vi "Physical Constant Menu.vi"() -> ()   [LabVIEW 2013]
panel:
  in  "Minimum Z Extension (nm)":dbl
  in  "Maximum Z Extension (nm)":dbl
  in  "Z Piezo Response (nm/V)":dbl
  in  "Minimum Y Extension (nm)":dbl
  in  "Maximum Y Extension (nm)":dbl
  in  "Y Piezo Response (nm/V)":dbl
  in  "Minimum X Extension (nm)":dbl
  in  "Maximum X Extension (nm)":dbl
  in  "X Piezo Response (nm/V)":dbl
  in  "Minimum Output Voltage (V)":dbl
  in  "Maximum Output Voltage (V)":dbl
  in  "Minimum Input Voltage (V)":dbl
  in  "Maximum Input Voltage (V)":dbl
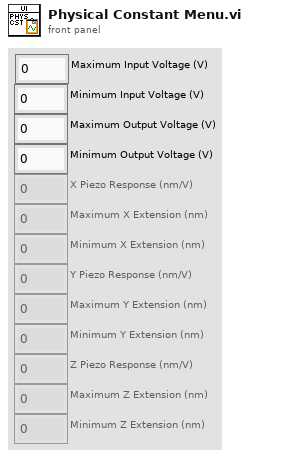
[diagram p1: front panel]
types:
  T1 = enum8{"Enabled", "Disabled", "Disabled and Grayed Out"}
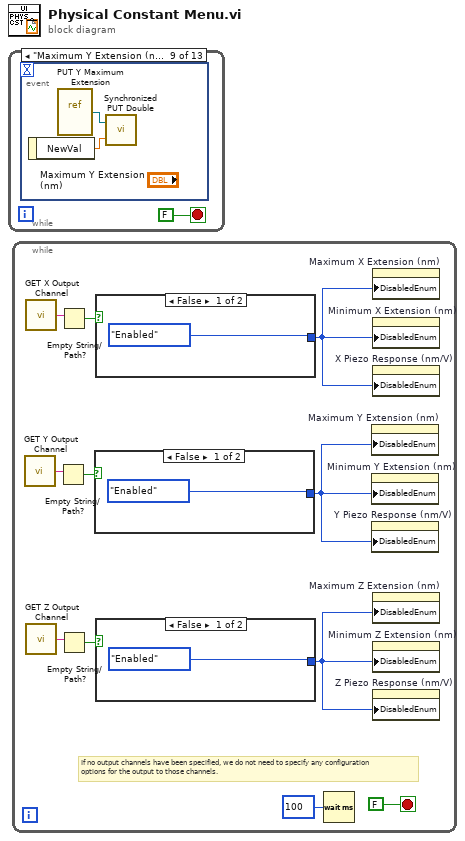
[diagram p0: block diagram]
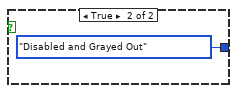
[diagram p2: hidden frame]
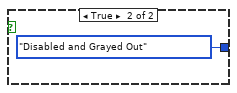
[diagram p3: hidden frame]
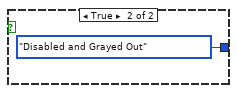
[diagram p4: hidden frame]
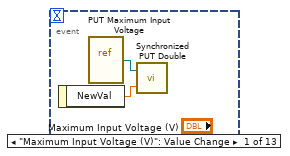
[diagram p5: hidden frame]
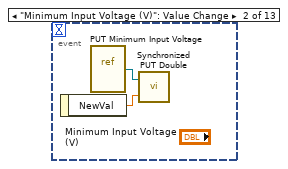
[diagram p6: hidden frame]
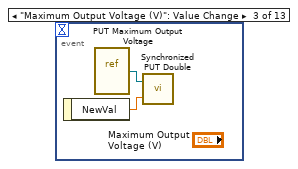
[diagram p7: hidden frame]
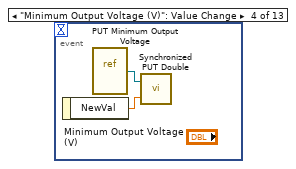
[diagram p8: hidden frame]
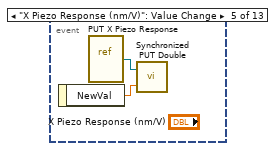
[diagram p9: hidden frame]
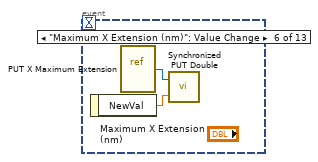
[diagram p10: hidden frame]
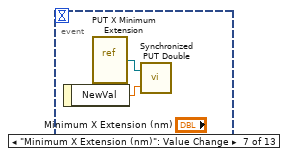
[diagram p11: hidden frame]
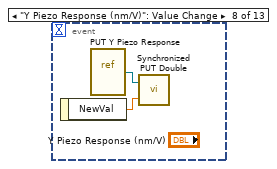
[diagram p12: hidden frame]
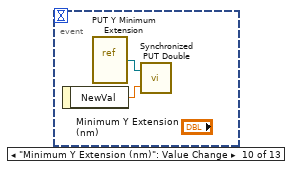
[diagram p13: hidden frame]
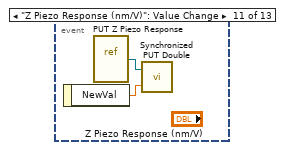
[diagram p14: hidden frame]
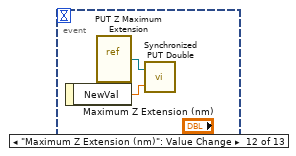
[diagram p15: hidden frame]
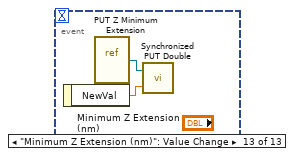
[diagram p16: hidden frame]
diagram:
  n1 = while {
    stop <- FALSE stop-if-true
    n2 = event shown="[8] \"Maximum Y Extension (nm)\": Value Change" {
      selector: _ -> [_ _ _ _ _ _ _ _ _ _ _ _ _]
      dyn-events: _ -> [_ _ _ _ _ _ _ _ _ _ _ _ _]
      timeout: _ -> [_ _ _ _ _ _ _ _ _ _ _ _ _]
      event "Maximum Input Voltage (V)": Value Change {
        n3 = event-data() -> ("NewVal"=w2:dbl)  [unwired: 1 in]
        n4 = vi-ref "PUT Maximum Input Voltage.vi"() -> (w3:refnum<vi>)
        n5 = call "Synchronized PUT Double.vi"("PUT Value"=w2, "PUT VI Reference"=w3) -> ()  [unwired: 1 in]
      }
      event "Minimum Input Voltage (V)": Value Change {
        n6 = event-data() -> ("NewVal"=w4:dbl)  [unwired: 1 in]
        n7 = vi-ref "PUT Minimum Input Voltage.vi"() -> (w5:refnum<vi>)
        n8 = call "Synchronized PUT Double.vi"("PUT Value"=w4, "PUT VI Reference"=w5) -> ()  [unwired: 1 in]
      }
      event "Maximum Output Voltage (V)": Value Change {
        n9 = event-data() -> ("NewVal"=w6:dbl)  [unwired: 1 in]
        n10 = vi-ref "PUT Maximum Output Voltage.vi"() -> (w7:refnum<vi>)
        n11 = call "Synchronized PUT Double.vi"("PUT Value"=w6, "PUT VI Reference"=w7) -> ()  [unwired: 1 in]
      }
      event "Minimum Output Voltage (V)": Value Change {
        n12 = event-data() -> ("NewVal"=w8:dbl)  [unwired: 1 in]
        n13 = vi-ref "PUT Minimum Output Voltage.vi"() -> (w9:refnum<vi>)
        n14 = call "Synchronized PUT Double.vi"("PUT Value"=w8, "PUT VI Reference"=w9) -> ()  [unwired: 1 in]
      }
      event "X Piezo Response (nm/V)": Value Change {
        n15 = event-data() -> ("NewVal"=w10:dbl)  [unwired: 1 in]
        n16 = vi-ref "PUT X Piezo Response.vi"() -> (w11:refnum<vi>)
        n17 = call "Synchronized PUT Double.vi"("PUT Value"=w10, "PUT VI Reference"=w11) -> ()  [unwired: 1 in]
      }
      event "Maximum X Extension (nm)": Value Change {
        n18 = event-data() -> ("NewVal"=w12:dbl)  [unwired: 1 in]
        n19 = vi-ref "PUT X Maximum Extension.vi"() -> (w13:refnum<vi>)
        n20 = call "Synchronized PUT Double.vi"("PUT Value"=w12, "PUT VI Reference"=w13) -> ()  [unwired: 1 in]
      }
      event "Minimum X Extension (nm)": Value Change {
        n21 = event-data() -> ("NewVal"=w14:dbl)  [unwired: 1 in]
        n22 = vi-ref "PUT X Minimum Extension.vi"() -> (w15:refnum<vi>)
        n23 = call "Synchronized PUT Double.vi"("PUT Value"=w14, "PUT VI Reference"=w15) -> ()  [unwired: 1 in]
      }
      event "Y Piezo Response (nm/V)": Value Change {
        n24 = event-data() -> ("NewVal"=w16:dbl)  [unwired: 1 in]
        n25 = vi-ref "PUT Y Piezo Response.vi"() -> (w17:refnum<vi>)
        n26 = call "Synchronized PUT Double.vi"("PUT Value"=w16, "PUT VI Reference"=w17) -> ()  [unwired: 1 in]
      }
      event "Maximum Y Extension (nm)": Value Change {
        n27 = event-data() -> ("NewVal"=w18:dbl)  [unwired: 1 in]
        n28 = vi-ref "PUT Y Maximum Extension.vi"() -> (w19:refnum<vi>)
        n29 = call "Synchronized PUT Double.vi"("PUT Value"=w18, "PUT VI Reference"=w19) -> ()  [unwired: 1 in]
      }
      event "Minimum Y Extension (nm)": Value Change {
        n30 = event-data() -> ("NewVal"=w20:dbl)  [unwired: 1 in]
        n31 = vi-ref "PUT Y Minimum Extension.vi"() -> (w21:refnum<vi>)
        n32 = call "Synchronized PUT Double.vi"("PUT Value"=w20, "PUT VI Reference"=w21) -> ()  [unwired: 1 in]
      }
      event "Z Piezo Response (nm/V)": Value Change {
        n33 = event-data() -> ("NewVal"=w22:dbl)  [unwired: 1 in]
        n34 = vi-ref "PUT Z Piezo Response.vi"() -> (w23:refnum<vi>)
        n35 = call "Synchronized PUT Double.vi"("PUT Value"=w22, "PUT VI Reference"=w23) -> ()  [unwired: 1 in]
      }
      event "Maximum Z Extension (nm)": Value Change {
        n36 = event-data() -> ("NewVal"=w24:dbl)  [unwired: 1 in]
        n37 = vi-ref "PUT Z Maximum Extension.vi"() -> (w25:refnum<vi>)
        n38 = call "Synchronized PUT Double.vi"("PUT Value"=w24, "PUT VI Reference"=w25) -> ()  [unwired: 1 in]
      }
      event "Minimum Z Extension (nm)": Value Change {
        n39 = event-data() -> ("NewVal"=w26:dbl)  [unwired: 1 in]
        n40 = vi-ref "PUT Z Minimum Extension.vi"() -> (w27:refnum<vi>)
        n41 = call "Synchronized PUT Double.vi"("PUT Value"=w26, "PUT VI Reference"=w27) -> ()  [unwired: 1 in]
      }
    }
  }
  n42 = while {
    stop <- FALSE stop-if-true
    # "If no output channels have been specified, we do not need to specify any configuration\noptions for the output to those channels."
    n43 = call "GET Y Output Channel.vi"() -> ("Y Output Channel"=w33:string)
    n44 = call "GET X Output Channel.vi"() -> ("X Output Channel"=w30:string)
    n45 = call "GET Z Output Channel.vi"() -> ("Z Output Channel"=w36:string)
    n46 = Empty String/Path?(string/path=w33) -> (empty?=w34:bool)
    n47 = Empty String/Path?(string/path=w30) -> (empty?=w31:bool)
    n48 = Empty String/Path?(string/path=w36) -> (empty?=w37:bool)
    n49 = case shown="False" w34 {
      tunnel: [T1."Enabled" ("Disabled") T1."Disabled and Grayed Out" ("Disabled")] -> w35
      frame False {
      }
      frame True {
      }
    }
    n50 = case shown="False" w31 {
      tunnel: [T1."Enabled" ("Disabled") T1."Disabled and Grayed Out" ("Disabled")] -> w32
      frame False {
      }
      frame True {
      }
    }
    n51 = case shown="False" w37 {
      tunnel: [T1."Enabled" ("Disabled") T1."Disabled and Grayed Out" ("Disabled")] -> w38
      frame False {
      }
      frame True {
      }
    }
    n52 = Wait (ms)(milliseconds to wait=u32 100) -> ()  [unwired: 1 out]
    n53 = property on="Maximum Y Extension (nm)" class="DigNum (strict)"("DisabledEnum"=w35) -> ()  [unwired: 2 in, 2 out]
    n54 = property on="Minimum Y Extension (nm)" class="DigNum (strict)"("DisabledEnum"=w35) -> ()  [unwired: 2 in, 2 out]
    n55 = property on="Y Piezo Response (nm/V)" class="DigNum (strict)"("DisabledEnum"=w35) -> ()  [unwired: 2 in, 2 out]
    n56 = property on="Maximum X Extension (nm)" class="DigNum (strict)"("DisabledEnum"=w32) -> ()  [unwired: 2 in, 2 out]
    n57 = property on="Minimum X Extension (nm)" class="DigNum (strict)"("DisabledEnum"=w32) -> ()  [unwired: 2 in, 2 out]
    n58 = property on="X Piezo Response (nm/V)" class="DigNum (strict)"("DisabledEnum"=w32) -> ()  [unwired: 2 in, 2 out]
    n59 = property on="Maximum Z Extension (nm)" class="DigNum (strict)"("DisabledEnum"=w38) -> ()  [unwired: 2 in, 2 out]
    n60 = property on="Minimum Z Extension (nm)" class="DigNum (strict)"("DisabledEnum"=w38) -> ()  [unwired: 2 in, 2 out]
    n61 = property on="Z Piezo Response (nm/V)" class="DigNum (strict)"("DisabledEnum"=w38) -> ()  [unwired: 2 in, 2 out]
  }
